vi "Home Reference.vi"(8 "Error in":errorcluster, 11 "Sample Test Template in":refnum<class "Sample Test Template.lvclass">) -> (0 "Error out":errorcluster, 2 "VI Ref":refnum<vi>, 3 "Sample Test Template out":refnum<class "Sample Test Template.lvclass">)   [LabVIEW 2020, in "Sample Test Template.lvclass"]
doc: "Dynamic method for status page reference"
uses:
  Sample Test Template.lvclass
  Parent/Typedef/LV2 Control.ctl
  Home Page.vi
  Parent/Test.lvclass
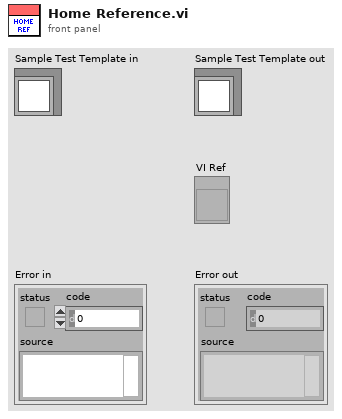
[diagram p1: front panel]
types:
  T1 = typedef "Test.lvclass/LV2 Control.ctl" = enum16{"Home", "Mode", "Config", "Status", "Read"}
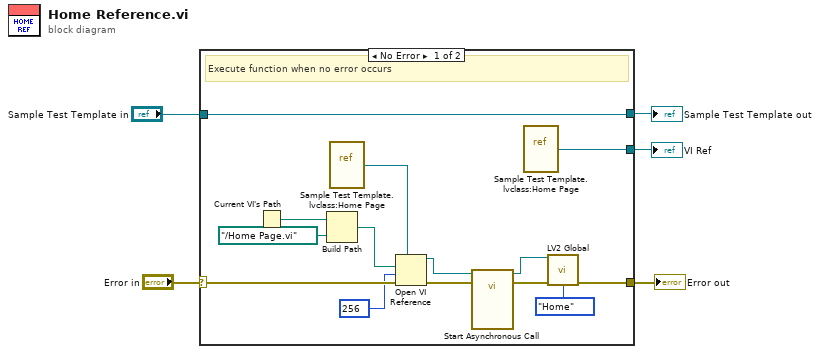
[diagram p0: block diagram]
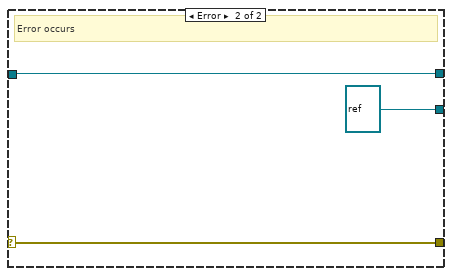
[diagram p2: hidden frame]
diagram:
  n1 = case shown="No Error" "Error in" {
    selector: "Error in" -> [w18 w22]
    tunnel: [w8 w22] -> w2
    tunnel: [w19 refnum<vi> refnum] -> w3
    tunnel: [w10 w20] -> w4
    tunnel: "Sample Test Template in" -> [w10 w20]
    frame No Error {
      # "Execute function when no error occurs"
      n2 = Current VI's Path() -> (path=w17:path)
      n3 = Build Path(base path=w17, name or relative path=path "../Home Page.vi") -> (appended path=w15:path)
      n4 = vi-ref "Sample Test Template.lvclass:Home Page.vi"() -> (w14:refnum<vi>)
      n5 = Open VI Reference(type specifier VI Refnum (for type only)=w14, vi path=w15, options=256, error in (no error)=w18) -> (vi reference=w13:refnum<vi>, error out=w12:errorcluster)  [unwired: 2 in]
      n6 = call-by-ref "Start Asynchronous Call"(reference=w13, error in=w12) -> (reference out=w6:refnum<vi>, error out=w9:errorcluster)  [unwired: 14 in, 2 out]
      n7 = vi-ref "Sample Test Template.lvclass:Home Page.vi"() -> (w19:refnum<vi>)
      n8 = call "LV2 Global.vi"("Home Ref In"=w6, "Error In"=w9, "Enum"=LV2_Control."Home") -> ("Error Out"=w8:errorcluster)  [unwired: 8 in, 4 out]
    }
    frame Error {
      # "Error occurs"
    }
  }
  "Error out" <- w2
  "Sample Test Template out" <- w4
  "VI Ref" <- w3
